vi "SetUp.vi"(8 "error in (no error)":errorcluster, 11 "Prueba04 in":refnum<class "Prueba04.lvclass">) -> (0 "error out":errorcluster, 3 "Prueba04 out":refnum<class "Prueba04.lvclass">)   [LabVIEW 2019, in "Prueba04.lvclass"]
uses:
  Prueba04.lvclass
  Prueba04.lvclass/Prueba04.ctl
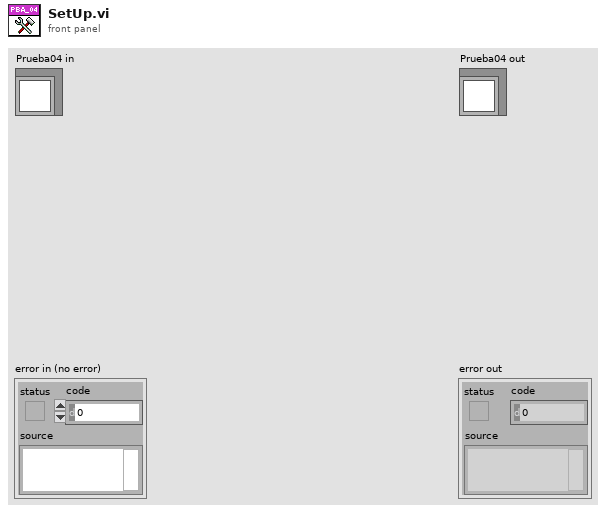
[diagram p1: front panel]
types:
  T1 = typedef "Prueba04.lvclass/BD.ctl" = cluster{"frec_referencia":dbl, "niv_presion_son_ref":dbl, "RangoMaxRef(dB)":dbl, "Incertidumbre":string[], "Tol +":string[], "Tol -":string[], "Frecuencias(Hz)":string[], "vol_enviado_CAM":dbl, "Ponderaciones A":dbl[], "Ponderaciones C":dbl[], "Ponderaciones Z":dbl[]}
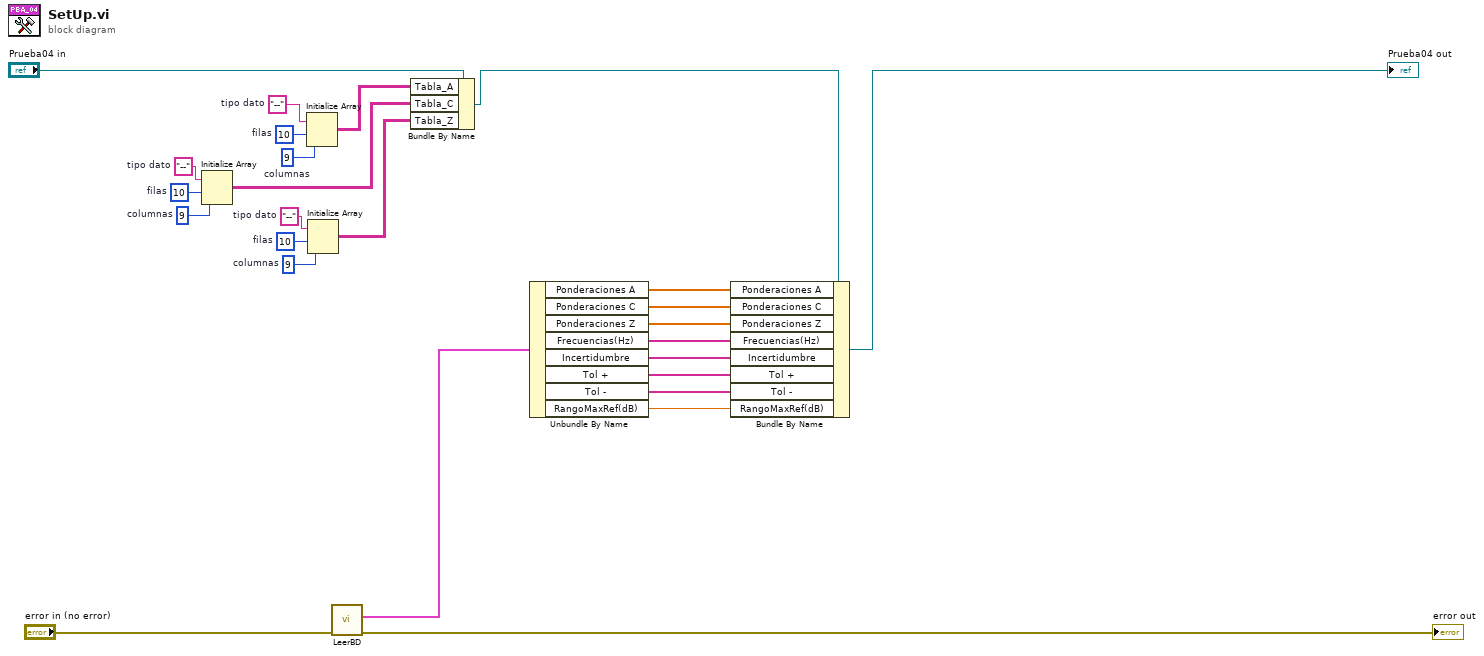
[diagram p0: block diagram]
diagram:
  w24 = 9  # columnas
  w25 = 10  # filas
  w23 = "--"  # tipo dato
  w21 = 9  # columnas
  w20 = 10  # filas
  w22 = "--"  # tipo dato
  w18 = 9  # columnas
  w19 = 10  # filas
  w17 = "--"  # tipo dato
  n1 = Initialize Array(w22, w20, w21) -> (w15:string[][])
  n2 = Initialize Array(w17, w19, w18) -> (w16:string[][])
  n3 = Initialize Array(w23, w25, w24) -> (w14:string[][])
  n4 = call "LeerBD.vi"("error in (no error)"="error in (no error)") -> ("error out"=→"error out":errorcluster, "BD"=w11:T1)  [unwired: 8 in, 1 out]
  n5 = Bundle By Name(cluster="Prueba04 in", "Tabla_A"=w16, "Tabla_C"=w15, "Tabla_Z"=w14) -> (w10:refnum<class "Prueba04.lvclass">)
  n6 = Unbundle By Name(w11) -> ("Ponderaciones A"=w3:dbl[], "Ponderaciones C"=w2:dbl[], "Ponderaciones Z"=w1:dbl[], "Frecuencias(Hz)"=w8:string[], "Incertidumbre"=w7:string[], "Tol +"=w6:string[], "Tol -"=w5:string[], "RangoMaxRef(dB)"=w4:dbl)
  n7 = Bundle By Name(cluster=w10, "Ponderaciones A"=w3, "Ponderaciones C"=w2, "Ponderaciones Z"=w1, "Frecuencias(Hz)"=w8, "Incertidumbre"=w7, "Tol +"=w6, "Tol -"=w5, "RangoMaxRef(dB)"=w4) -> (→"Prueba04 out":refnum<class "Prueba04.lvclass">)
